vi "About.vi"   [LabVIEW 2020]
panel:
  # "iRho-100型反应性仪 v3.0.1\n\n版权所有：2021 核星核电科技(海盐)有限公司                www.nustarnuclear.com"
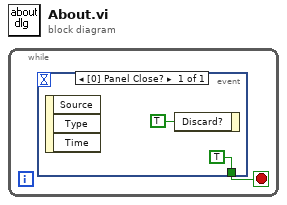
[diagram p0: block diagram]
diagram:
  n1 = while {
    stop <- w1 stop-if-true
    n2 = event shown="[0] Panel Close?" {
      selector: _ -> [_]
      dyn-events: _ -> [_]
      timeout: _ -> [_]
      tunnel: [TRUE ("Discard?")] -> w1
      event Panel Close? {
        n3 = event-data() -> ()  [unwired: 1 in, 3 out]
        n4 = event-data("Discard?"=TRUE) -> ()  [unwired: 1 in, 1 out]
      }
    }
  }
